vi "Float32_conv_1 (SubVI).vi"(11 "data in":string) -> (2 "data out":sgl[](array[numeric]))   [LabVIEW 2015]
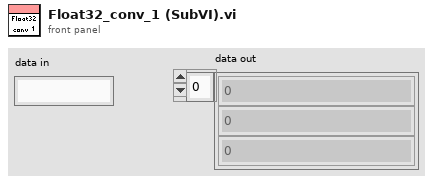
[diagram p1: front panel]
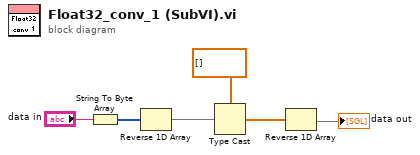
[diagram p0: block diagram]
diagram:
  n1 = String To Byte Array(string="data in") -> (unsigned byte array=w5:u8[])
  n2 = Reverse 1D Array(array=w5) -> (reversed array=w2:u8[])
  n3 = Type Cast(type=sgl[] [], x=w2) -> (*(type *) &x=w1:sgl[])
  n4 = Reverse 1D Array(array=w1) -> (reversed array=→"data out":sgl[])
